vi "Update Created.vi"(6 "Labels":map{string, string}(c390), 8 "error in (no error)":errorcluster, 11 "Counter in":refnum<class "Counter.lvclass">) -> (0 "error out":errorcluster, 3 "Counter out":refnum<class "Counter.lvclass">)   [LabVIEW 2020, in "Metrics.lvlib" / "Counter.lvclass"]
uses:
  Counter.lvclass
  Counter.lvclass/Counter.ctl
  metric/Metric.lvclass
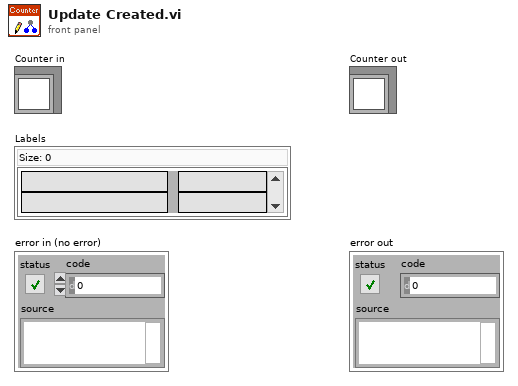
[diagram p1: front panel]
types:
  T1 = enum16{"seconds", "milliseconds", "microseconds"}
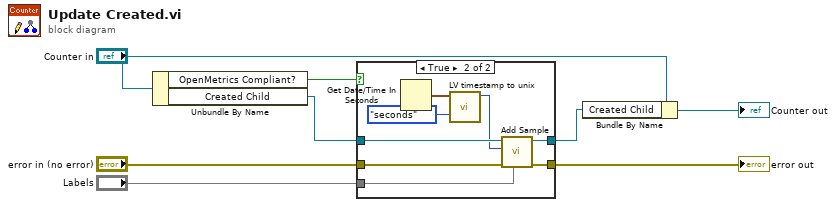
[diagram p0: block diagram]
diagram:
  n1 = Unbundle By Name("Counter in") -> ("OpenMetrics Compliant?"=w1:bool, "Created Child"=w2:refnum<class "Metric.lvclass">)
  n2 = case shown="True" w1 {
    tunnel: w2 -> [w10 w18]
    tunnel: "Labels" -> [_ w14]
    tunnel: [w10 w13] -> w5
    tunnel: "error in (no error)" -> [w9 w11]
    tunnel: [w9 w12] -> w8
    frame False {
    }
    frame True {
      n3 = Get Date/Time In Seconds() -> (seconds since 1Jan1904=w17:timestamp)
      n4 = call "LV timestamp to unix.vi"("Precision (ms)"=T1."seconds", "Timestamp"=w17) -> ("Unix epoch time"=w15:u64)  [unwired: 9 in]
      n5 = call-dynamic "Add Sample.vi"("Labels"=w14, "error in (no error)"=w11, "Value"=w15, "Metric in"=w18) -> ("error out"=w12:errorcluster, "Metric out"=w13:refnum<class "Metric.lvclass">)  [unwired: 6 in]
    }
  }
  "error out" <- w8
  n6 = Bundle By Name(cluster="Counter in", "Created Child"=w5) -> (→"Counter out":refnum<class "Counter.lvclass">)
